vi "Initialize Bus Monitor.vi"(8 "error in (no error)":errorcluster, 11 "ListboxBusMonitor In":refnum<class "ListboxBusMonitor.lvclass">) -> (0 "error out":errorcluster, 3 "ListboxBusMonitor Out":refnum<class "ListboxBusMonitor.lvclass">)   [LabVIEW 2017, in "ListboxBusMonitor.lvlib" / "ListboxBusMonitor.lvclass"]
uses:
  ListboxBusMonitor.lvclass
  ListboxBusMonitor.lvclass/ListboxBusMonitor.ctl
  ListboxBusMonitorPanel/ListboxBusMonitorPanel.lvclass/ListboxBusMonitorPanel.ctl
  ListboxBusMonitorPanel/ListboxBusMonitorPanel.lvclass
  C:/Program Files (x86)/National Instruments/LabVIEW 2017/vi.lib/ActorFramework/Actor/Actor.lvclass
  <vilib>/ActorFramework/Actor/Actor.lvclass
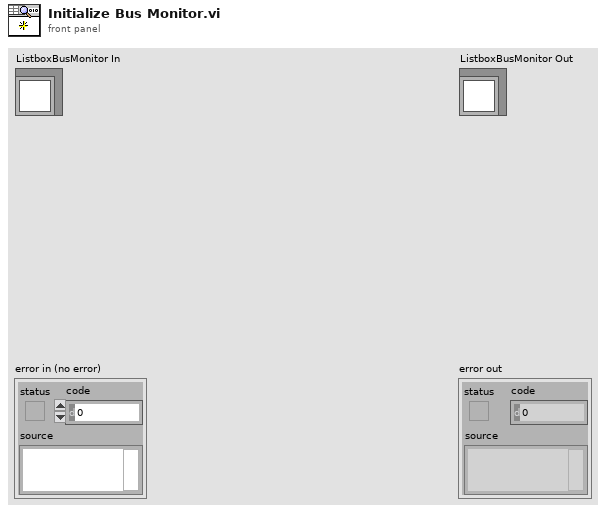
[diagram p1: front panel]
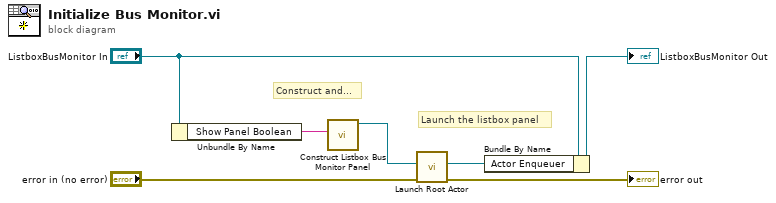
[diagram p0: block diagram]
diagram:
  # "Construct and..."
  # "Launch the listbox panel"
  n1 = Unbundle By Name("ListboxBusMonitor In") -> ("Show Panel Boolean"=w1:string)
  n2 = call "Construct Listbox Bus Monitor Panel.vi"("Show Panel Boolean"=w1) -> ("ListboxBusMonitorPanel out"=w3:refnum<class "ListboxBusMonitorPanel.lvclass">)  [unwired: 10 in]
  n3 = call <vilib>:"Launch Root Actor.vi"("error in (no error)"="error in (no error)", "Actor"=w3) -> ("error out"=→"error out":errorcluster, "Actor's Enqueuer"=w4:refnum<class "Message Enqueuer.lvclass">)  [unwired: 8 in]
  n4 = Bundle By Name(cluster="ListboxBusMonitor In", "Actor Enqueuer"=w4) -> (→"ListboxBusMonitor Out":refnum<class "ListboxBusMonitor.lvclass">)
